vi "Set Voltage.vi"(8 "error in (no error)":errorcluster, 10 "Voltage":dbl, 11 "Simulated PSU in":refnum<class "Simulated PSU.lvclass">) -> (0 "error out":errorcluster, 3 "Simulated PSU out":refnum<class "Simulated PSU.lvclass">)   [LabVIEW 2020, in "Simulated PSU.lvlib" / "Simulated PSU.lvclass"]
uses:
  Simulated PSU.lvclass
  Simulated PSU.lvclass/Simulated PSU.ctl
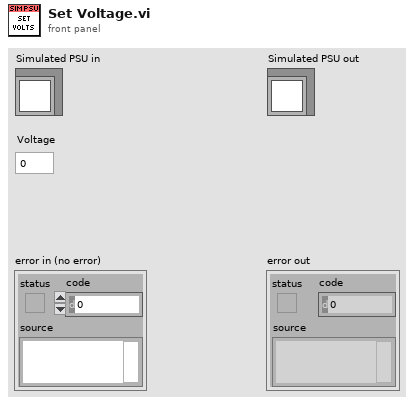
[diagram p1: front panel]
types:
  T1 = typedef "Simulated PSU.lvlib/Simulated PSU.lvclass/Ref Data.ctl" = cluster{"Enabled":bool, "Voltage":dbl, "Noise Level":dbl, "Resistance":dbl}
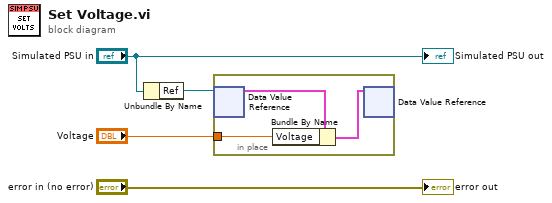
[diagram p0: block diagram]
diagram:
  n1 = Unbundle By Name("Simulated PSU in") -> ("Ref"=w3:refnum<data-value>)
  n2 = in-place {
    in-place-border: "Voltage" -> [w5]
    n3 = in-place-dvr #1(w3) -> (w7:T1)  [unwired: 1 out]
    n4 = Bundle By Name(cluster=w7, "Voltage"=w5) -> (w6:T1)
    n5 = in-place-dvr #1(w6) -> ()  [unwired: 2 out]
  }
  "error out" <- "error in (no error)"
  "Simulated PSU out" <- "Simulated PSU in"
